vi "Read Handle.vi"(8 "Error In":errorcluster, 11 "Known Host In":refnum<class "KnownHost.lvclass">) -> (0 "Erorr Out":errorcluster, 2 "Handle":u64, 3 "Known Host Out":refnum<class "KnownHost.lvclass">)   [LabVIEW 2017, in "Toolkit.lvlib" / "KnownHost.lvclass"]
uses:
  KnownHost.lvclass
  KnownHost.lvclass/KnownHost.ctl
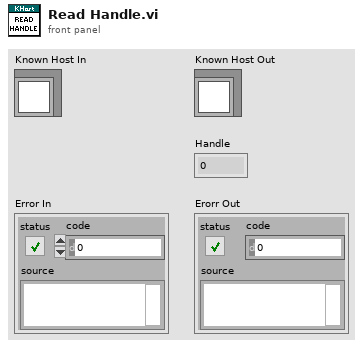
[diagram p1: front panel]
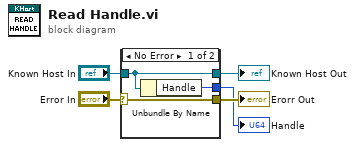
[diagram p0: block diagram]
diagram:
  n1 = case shown="No Error" "Error In" {
    selector: "Error In" -> [w8 w9]
    tunnel: [w8 w9] -> w4
    tunnel: "Known Host In" -> [w7 w10]
    tunnel: [w7 w10] -> w1
    tunnel: [w6 _] -> w3
    frame No Error {
      n2 = Unbundle By Name(w7) -> ("Handle"=w6:u64)
    }
    frame Error {
    }
  }
  "Erorr Out" <- w4
  "Handle" <- w3
  "Known Host Out" <- w1
